vi "String Constant - Through Nested Case Structure.vi"() -> ()   [LabVIEW 2020]
panel:
  in  "OK":bool
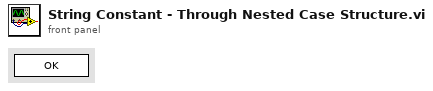
[diagram p1: front panel]
types:
  T1 = enum32{"Invalid", "Standard", "Closed", "Hidden", "Minimized", "Maximized"}
  T2 = enum32{"invalid app kind", "Development System", "Run Time System", "Student Edition", "Embedded LabVIEW", "Evaluation", "Custom"}
  T3 = cluster{"Core":cluster{"Current VI Reference":refnum<vi>, "Close Panel on Exit?":bool}, "Your Boolean data":bool}
  T4 = cluster{"Current VI Reference":refnum<vi>, "Close Panel on Exit?":bool}
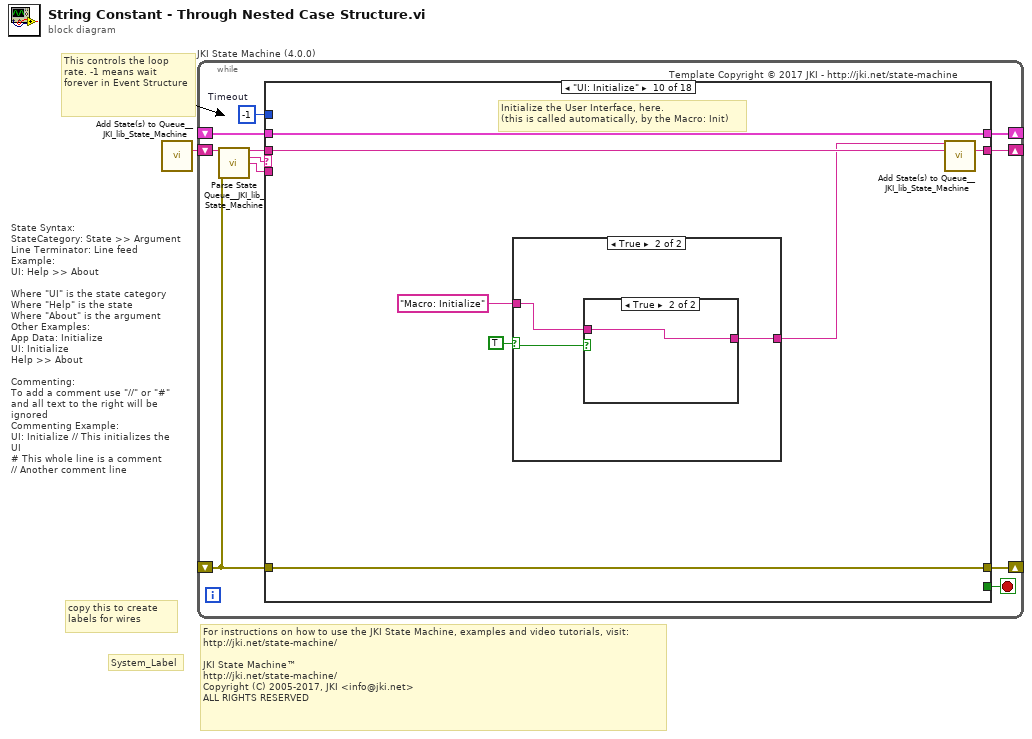
[diagram p0: block diagram]
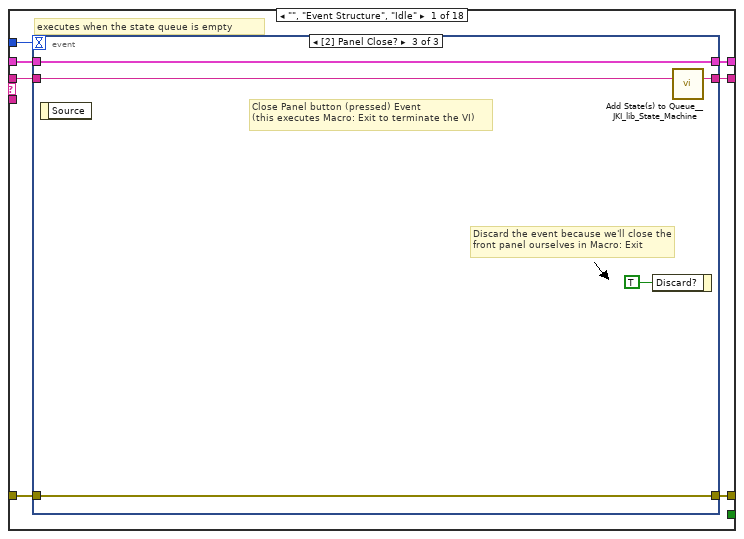
[diagram p2: hidden frame]
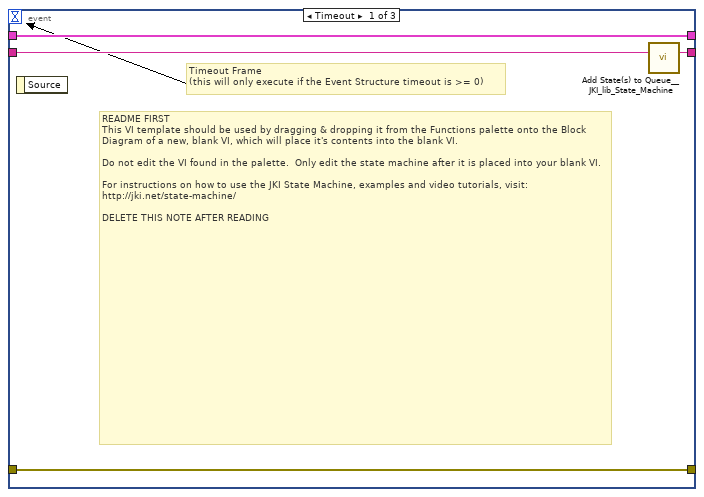
[diagram p3: hidden frame]
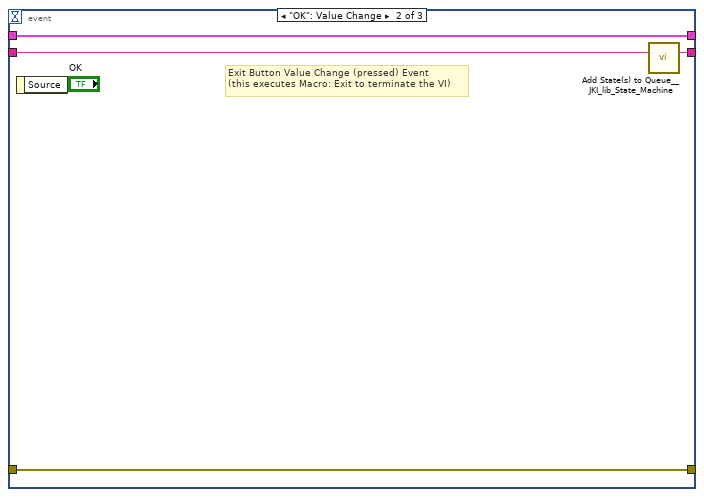
[diagram p4: hidden frame]
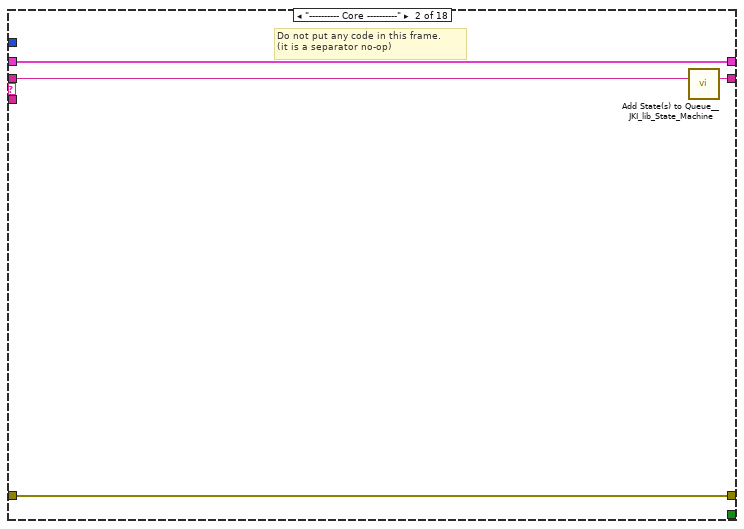
[diagram p5: hidden frame]
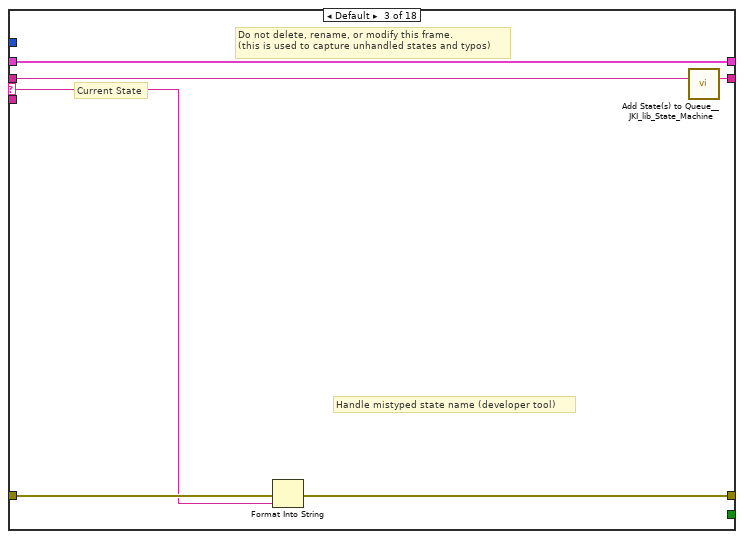
[diagram p6: hidden frame]
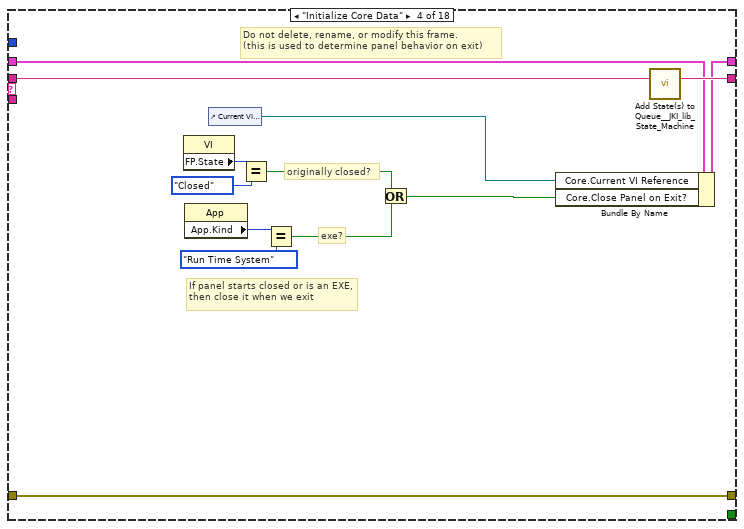
[diagram p7: hidden frame]
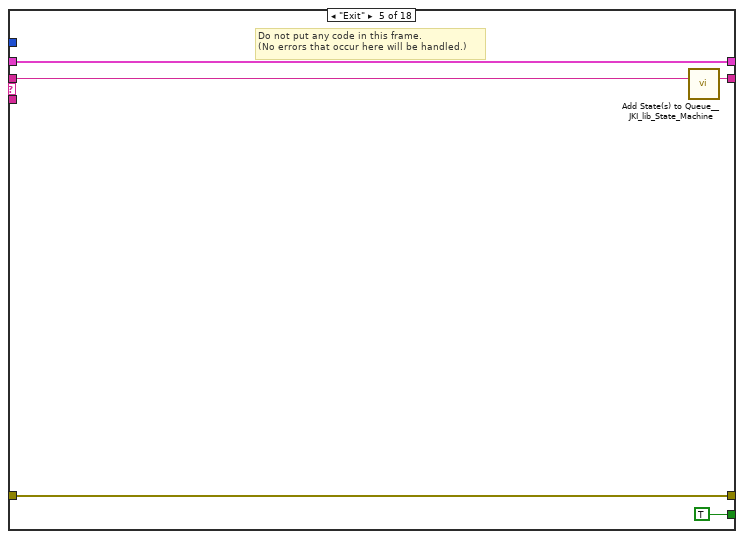
[diagram p8: hidden frame]
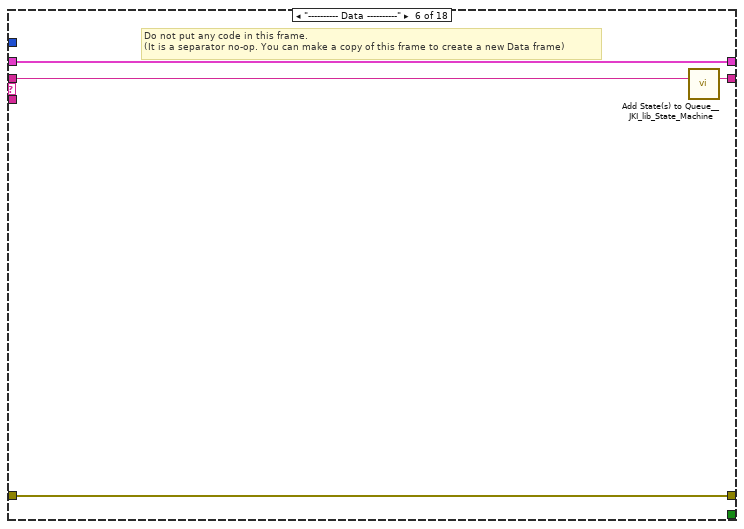
[diagram p9: hidden frame]
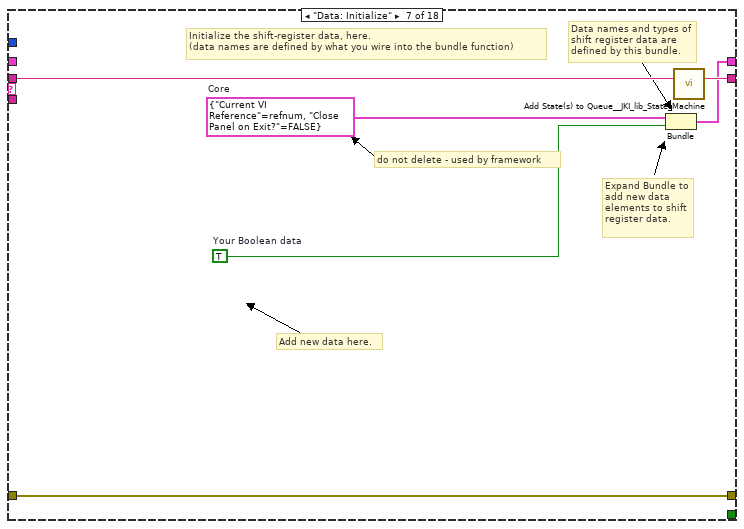
[diagram p10: hidden frame]
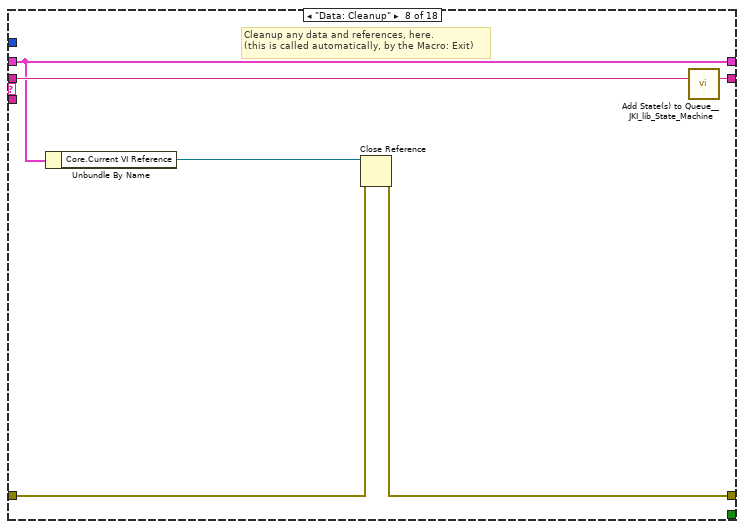
[diagram p11: hidden frame]
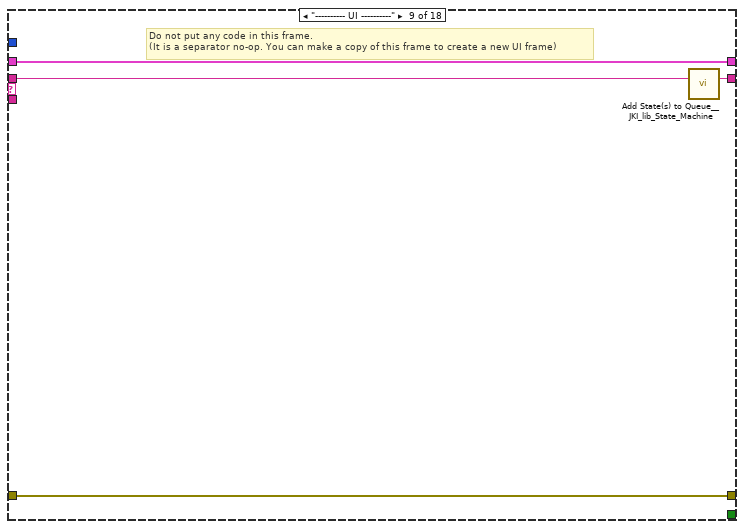
[diagram p12: hidden frame]
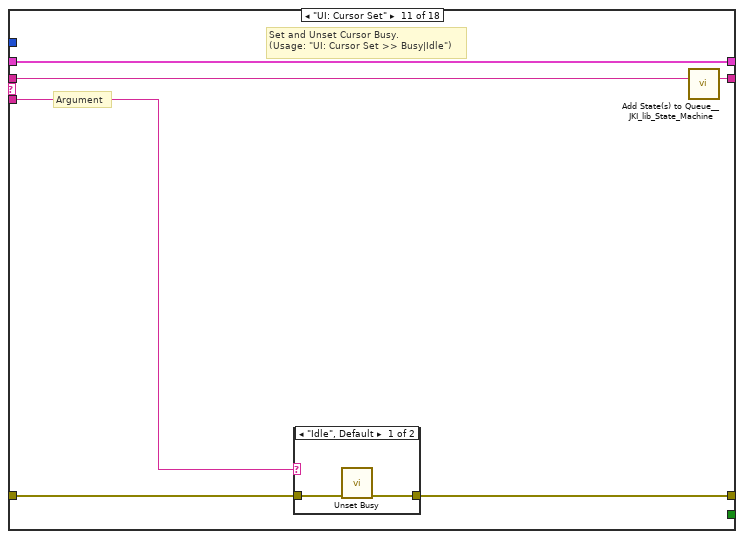
[diagram p15: hidden frame]
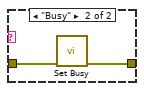
[diagram p16: hidden frame]
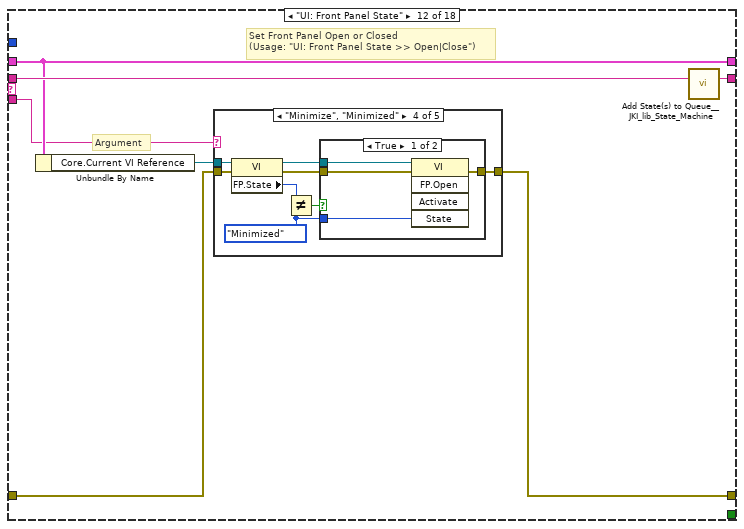
[diagram p17: hidden frame]
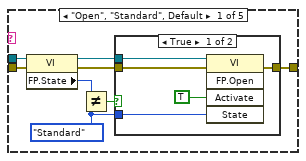
[diagram p18: hidden frame]
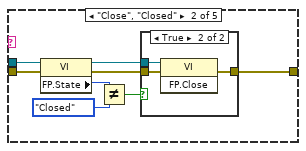
[diagram p20: hidden frame]
diagram:
  # "For instructions on how to use the JKI State Machine, examples and video tutorials, visit:\nhttp://jki.net/state-machine/\n\nJKI State Machine™\nhttp://jki.net/state-machine/\nCopyright (C) 2005-2017, JKI <info@jki.net>\nALL RIGHTS RESERVED"
  # "State Syntax:\nStateCategory: State >> Argument\nLine Terminator: Line feed\nExample:\nUI: Help >> About\n\nWhere \"UI\" is the state category\nWhere \"Help\" is the state\nWhere \"About\" is the argument\nOther Examples:\nApp Data: Initialize\nUI: Initialize\nHelp >> About\n\nCommenting:\nTo add a comment use \"//\" or \"#\" and all text to the right will be ignored\nCommenting Example:\nUI: Initialize // This initializes the UI\n# This whole line is a comment\n// Another comment line"
  # "copy this to create labels for wires"
  # "This controls the loop rate. -1 means wait forever in Event Structure"
  # "System_Label"
  n1 = call <vilib>:"Add State(s) to Queue__JKI_lib_State_Machine.vi"() -> ("States Out"=w1:string)  [unwired: 15 in]
  n2 = while "JKI State Machine (4.0.0)" {
    shift-right: [w5] -> _
    shift-left: _ -> [w4]
    shift-right: [w8] -> _
    shift-left: _ -> [w2]
    shift-right: [w7] -> _
    shift-left: w1 -> [w9]
    stop <- w6 stop-if-true
    w3 = -1  # Timeout
    # "Template Copyright © 2017 JKI - http://jki.net/state-machine"
    n3 = call <vilib>:"Parse State Queue__JKI_lib_State_Machine.vi"("State Queue"=w9, "Error In (no error)"=w2) -> ("Remaining States"=w11:string, "Current State"=w12:string, "Arguments"=w10:string)  [unwired: 11 in]
    n4 = case shown="\"UI: Initialize\"" w12 {
      selector: w12 -> [_ _ w37 _ _ _ _ _ _ _ _ _ _ _ _ _ _ _]
      tunnel: w11 -> [w19 w36 w40 w55 w60 w64 w70 w76 w80 w87 w97 w108 w177 w181 w185 w189 w193 w197]
      tunnel: w10 -> [_ _ _ _ _ _ _ _ _ _ w92 w102 _ _ _ _ _ _]
      tunnel: w4 -> [w17 w33 w38 w48 w58 w61 _ w71 w77 w85 w95 w104 w174 w178 w182 w186 w190 w194]
      tunnel: [w16 w34 w42 w52 w57 w62 w67 w72 w78 w84 w93 w105 w175 w179 w183 w187 w191 w195] -> w8
      tunnel: w2 -> [w15 w34 w41 w52 w57 w62 w67 w73 w78 w84 w94 w106 w175 w179 w183 w187 w191 w195]
      tunnel: [w18 w35 w39 w54 w59 w63 w69 w75 w79 w86 w96 w107 w176 w180 w184 w188 w192 w196] -> w7
      tunnel: [_ _ _ _ TRUE _ _ _ _ _ _ _ _ _ _ _ _ _] -> w6
      tunnel: [w14 w33 w38 w53 w58 w61 w68 w71 w77 w85 w95 w104 w174 w178 w182 w186 w190 w194] -> w5
      tunnel: w3 -> [w13 _ _ _ _ _ _ _ _ _ _ _ _ _ _ _ _ _]
      frame "", "Event Structure", "Idle" {
        # "executes when the state queue is empty"
        n5 = event shown="[2] Panel Close?" {
          selector: _ -> [_ _ _]
          dyn-events: _ -> [_ _ _]
          timeout: w13 -> [_ _ _]
          tunnel: w19 -> [w23 w27 w32]
          tunnel: [w22 w26 w31] -> w18
          tunnel: w17 -> [w20 w24 w29]
          tunnel: [w21 w25 w30] -> w16
          tunnel: w15 -> [w21 w25 w30]
          tunnel: [w20 w24 w29] -> w14
          event Timeout {
            # "README FIRST\nThis VI template should be used by dragging & dropping it from the Functions palette onto the Block Diagram of a new, blank VI, which will place it's contents into the blank VI.\n\nDo not edit the VI found in the palette.  Only edit the state machine after it is placed into your blank VI.\n\nFor instructions on how to use the JKI State Machine, examples and video tutorials, visit:\nhttp://jki.net/state-machine/\n\nDELETE THIS NOTE AFTER READING"
            # "Timeout Frame\n(this will only execute if the Event Structure timeout is >= 0)"
            n6 = event-data() -> ()  [unwired: 1 in, 1 out]
            n7 = call <vilib>:"Add State(s) to Queue__JKI_lib_State_Machine.vi"("State(s) in (\"\")"=w23) -> ("States Out"=w22:string)  [unwired: 14 in]
          }
          event "OK": Value Change {
            # "Exit Button Value Change (pressed) Event\n(this executes Macro: Exit to terminate the VI)"
            n8 = event-data() -> ()  [unwired: 1 in, 1 out]
            n9 = call <vilib>:"Add State(s) to Queue__JKI_lib_State_Machine.vi"("State(s) in (\"\")"=w27) -> ("States Out"=w26:string)  [unwired: 14 in]
          }
          event Panel Close? {
            # "Discard the event because we'll close the front panel ourselves in Macro: Exit"
            # "Close Panel button (pressed) Event\n(this executes Macro: Exit to terminate the VI)"
            n10 = event-data() -> ()  [unwired: 1 in, 1 out]
            n11 = event-data("Discard?"=TRUE) -> ()  [unwired: 1 in, 1 out]
            n12 = call <vilib>:"Add State(s) to Queue__JKI_lib_State_Machine.vi"("State(s) in (\"\")"=w32) -> ("States Out"=w31:string)  [unwired: 14 in]
          }
        }
      }
      frame "---------- Core ----------" {
        # "Do not put any code in this frame.\n(it is a separator no-op)"
        n13 = call <vilib>:"Add State(s) to Queue__JKI_lib_State_Machine.vi"("State(s) in (\"\")"=w36) -> ("States Out"=w35:string)  [unwired: 14 in]
      }
      frame Default {
        # "Current State"
        # "Do not delete, rename, or modify this frame.\n(this is used to capture unhandled states and typos)"
        # "Handle mistyped state name (developer tool)"
        n14 = Format Into String(error in=w41, w37) -> (error out=w42:errorcluster)  [unwired: 2 in, 1 out]
        n15 = call <vilib>:"Add State(s) to Queue__JKI_lib_State_Machine.vi"("State(s) in (\"\")"=w40) -> ("States Out"=w39:string)  [unwired: 14 in]
      }
      frame "Initialize Core Data" {
        # "Do not delete, rename, or modify this frame.\n(this is used to determine panel behavior on exit)"
        # "originally closed?"
        # "exe?"
        # "If panel starts closed or is an EXE, then close it when we exit"
        n16 = property class="VI"() -> ("FP.State"=w45:T1)  [unwired: 2 in, 2 out]
        n17 = property class="App"() -> ("App.Kind"=w51:T2)  [unwired: 2 in, 2 out]
        n18 = control-ref of="Current VI Reference"() -> (w46:refnum<vi>)
        n19 = Equal?(x=w45, y=T1."Closed" ("Front Panel Window:State")) -> (x = y?=w43:bool)
        n20 = Equal?(x=w51, y=T2."Run Time System" ("Application:Kind")) -> (x = y?=w49:bool)
        n21 = Or(x=w43, y=w49) -> (x .or. y?=w47:bool)
        n22 = Bundle By Name(cluster=w48, "Core.Current VI Reference"=w46, "Core.Close Panel on Exit?"=w47) -> (w53:T3)
        n23 = call <vilib>:"Add State(s) to Queue__JKI_lib_State_Machine.vi"("State(s) in (\"\")"=w55) -> ("States Out"=w54:string)  [unwired: 14 in]
      }
      frame "Exit" {
        # "Do not put any code in this frame.\n(No errors that occur here will be handled.)"
        n24 = call <vilib>:"Add State(s) to Queue__JKI_lib_State_Machine.vi"("State(s) in (\"\")"=w60) -> ("States Out"=w59:string)  [unwired: 14 in]
      }
      frame "---------- Data ----------" {
        # "Do not put any code in this frame.\n(It is a separator no-op. You can make a copy of this frame to create a new Data frame)"
        n25 = call <vilib>:"Add State(s) to Queue__JKI_lib_State_Machine.vi"("State(s) in (\"\")"=w64) -> ("States Out"=w63:string)  [unwired: 14 in]
      }
      frame "Data: Initialize" {
        w65 = T4 {"Current VI Reference"=refnum, "Close Panel on Exit?"=FALSE}  # Core
        w66 = TRUE  # Your Boolean data
        # "do not delete - used by framework"
        # "Expand Bundle to add new data elements to shift register data."
        # "Add new data here."
        # "Data names and types of shift register data are defined by this bundle."
        # "Initialize the shift-register data, here.\n(data names are defined by what you wire into the bundle function)"
        n26 = Bundle("Core"=w65, "Your Boolean data"=w66) -> (w68:T3)  [unwired: 1 in]
        n27 = call <vilib>:"Add State(s) to Queue__JKI_lib_State_Machine.vi"("State(s) in (\"\")"=w70) -> ("States Out"=w69:string)  [unwired: 14 in]
      }
      frame "Data: Cleanup" {
        # "Cleanup any data and references, here.\n(this is called automatically, by the Macro: Exit)"
        n28 = Unbundle By Name(w71) -> ("Core.Current VI Reference"=w74:refnum<vi>)
        n29 = Close Reference(reference=w74, error in (no error)=w73) -> (error out=w72:errorcluster)
        n30 = call <vilib>:"Add State(s) to Queue__JKI_lib_State_Machine.vi"("State(s) in (\"\")"=w76) -> ("States Out"=w75:string)  [unwired: 14 in]
      }
      frame "---------- UI ----------" {
        # "Do not put any code in this frame.\n(It is a separator no-op. You can make a copy of this frame to create a new UI frame)"
        n31 = call <vilib>:"Add State(s) to Queue__JKI_lib_State_Machine.vi"("State(s) in (\"\")"=w80) -> ("States Out"=w79:string)  [unwired: 14 in]
      }
      frame "UI: Initialize" {
        # "Initialize the User Interface, here.\n(this is called automatically, by the Macro: Init)"
        n32 = case shown="True" TRUE {
          selector: TRUE -> [_ w89]
          tunnel: [_ w90] -> w83
          tunnel: "Macro: Initialize" -> [_ w88]
          frame False {
          }
          frame True {
            n33 = case shown="True" w89 {
              tunnel: [_ w91] -> w90
              tunnel: w88 -> [_ w91]
              frame False {
              }
              frame True {
              }
            }
          }
        }
        n34 = call <vilib>:"Add State(s) to Queue__JKI_lib_State_Machine.vi"("State(s) in Front (\"\")"=w83, "State(s) in (\"\")"=w87) -> ("States Out"=w86:string)  [unwired: 13 in]
      }
      frame "UI: Cursor Set" {
        # "Argument"
        # "Set and Unset Cursor Busy.\n(Usage: \"UI: Cursor Set >> Busy|Idle\")"
        n35 = case shown="\"Idle\", Default" w92 {
          tunnel: w94 -> [w99 w101]
          tunnel: [w98 w100] -> w93
          frame "Idle", Default {
            n36 = call <vilib>:"Unset Busy.vi"("error in (no error)"=w99) -> ("error out"=w98:errorcluster)  [unwired: 10 in]
          }
          frame "Busy" {
            n37 = call <vilib>:"Set Busy.vi"("error in (no error)"=w101) -> ("error out"=w100:errorcluster)  [unwired: 9 in, 1 out]
          }
        }
        n38 = call <vilib>:"Add State(s) to Queue__JKI_lib_State_Machine.vi"("State(s) in (\"\")"=w97) -> ("States Out"=w96:string)  [unwired: 14 in]
      }
      frame "UI: Front Panel State" {
        # "Argument"
        # "Set Front Panel Open or Closed\n(Usage: \"UI: Front Panel State >> Open|Close\")"
        n39 = Unbundle By Name(w104) -> ("Core.Current VI Reference"=w103:refnum<vi>)
        n40 = case shown="\"Minimize\", \"Minimized\"" w102 {
          tunnel: w106 -> [w114 w129 w140 w153 w166]
          tunnel: [w116 w130 w142 w155 w168] -> w105
          tunnel: w103 -> [w115 w127 w141 w154 w167]
          frame "Open", "Standard", Default {
            w109 = T1."Standard" ("State")
            n41 = property class="VI"(reference=w115, error in=w114) -> (reference out=w112:refnum<vi>, error out=w113:errorcluster, "FP.State"=w111:T1)
            n42 = Not Equal?(x=w111, y=w109) -> (x != y?=w110:bool)
            n43 = case shown="True" w110 {
              tunnel: [w120 w122] -> w116
              tunnel: w113 -> [w119 w122]
              tunnel: w112 -> [w118 _]
              tunnel: w109 -> [w117 _]
              frame True {
                n44 = invoke class="VI" method="FP.Open"(reference=w118, error in=w119, "Activate"=TRUE, "State"=w117) -> (error out=w120:errorcluster)  [unwired: 1 in, 4 out]
              }
              frame False {
              }
            }
          }
          frame "Close", "Closed" {
            n45 = property class="VI"(reference=w127, error in=w129) -> (reference out=w126:refnum<vi>, error out=w128:errorcluster, "FP.State"=w124:T1)
            n46 = Not Equal?(x=w124, y=T1."Closed" ("Front Panel Window:State")) -> (x != y?=w123:bool)
            n47 = case shown="True" w123 {
              tunnel: [w131 w134] -> w130
              tunnel: w128 -> [w131 w133]
              tunnel: w126 -> [_ w132]
              frame False {
              }
              frame True {
                n48 = invoke class="VI" method="FP.Close"(reference=w132, error in=w133) -> (error out=w134:errorcluster)  [unwired: 1 in, 2 out]
              }
            }
          }
          frame "Hidden", "Hide" {
            w135 = T1."Hidden" ("State")
            n49 = property class="VI"(reference=w141, error in=w140) -> (reference out=w138:refnum<vi>, error out=w139:errorcluster, "FP.State"=w137:T1)
            n50 = Not Equal?(x=w137, y=w135) -> (x != y?=w136:bool)
            n51 = case shown="True" w136 {
              tunnel: [w146 w147] -> w142
              tunnel: w139 -> [w145 w147]
              tunnel: w138 -> [w144 _]
              tunnel: w135 -> [w143 _]
              frame True {
                n52 = invoke class="VI" method="FP.Open"(reference=w144, error in=w145, "State"=w143) -> (error out=w146:errorcluster)  [unwired: 2 in, 4 out]
              }
              frame False {
              }
            }
          }
          frame "Minimize", "Minimized" {
            w148 = T1."Minimized" ("State")
            n53 = property class="VI"(reference=w154, error in=w153) -> (reference out=w151:refnum<vi>, error out=w152:errorcluster, "FP.State"=w150:T1)
            n54 = Not Equal?(x=w150, y=w148) -> (x != y?=w149:bool)
            n55 = case shown="True" w149 {
              tunnel: [w159 w160] -> w155
              tunnel: w152 -> [w158 w160]
              tunnel: w151 -> [w157 _]
              tunnel: w148 -> [w156 _]
              frame True {
                n56 = invoke class="VI" method="FP.Open"(reference=w157, error in=w158, "State"=w156) -> (error out=w159:errorcluster)  [unwired: 2 in, 4 out]
              }
              frame False {
              }
            }
          }
          frame "Maximize", "Maximized" {
            w161 = T1."Maximized" ("State")
            n57 = property class="VI"(reference=w167, error in=w166) -> (reference out=w164:refnum<vi>, error out=w165:errorcluster, "FP.State"=w163:T1)
            n58 = Not Equal?(x=w163, y=w161) -> (x != y?=w162:bool)
            n59 = case shown="True" w162 {
              tunnel: [w172 w173] -> w168
              tunnel: w165 -> [w171 w173]
              tunnel: w164 -> [w170 _]
              tunnel: w161 -> [w169 _]
              frame True {
                n60 = invoke class="VI" method="FP.Open"(reference=w170, error in=w171, "State"=w169) -> (error out=w172:errorcluster)  [unwired: 2 in, 4 out]
              }
              frame False {
              }
            }
          }
        }
        n61 = call <vilib>:"Add State(s) to Queue__JKI_lib_State_Machine.vi"("State(s) in (\"\")"=w108) -> ("States Out"=w107:string)  [unwired: 14 in]
      }
      frame "---------- Macro ----------" {
        # "Do not put any code in this frame.\n(It is a separator no-op. You can make a copy of this frame to create a new Macro frame)"
        n62 = call <vilib>:"Add State(s) to Queue__JKI_lib_State_Machine.vi"("State(s) in (\"\")"=w177) -> ("States Out"=w176:string)  [unwired: 14 in]
      }
      frame "Macro: Initialize" {
        # "Initialization Macro\n(This is called once, when the VI starts)"
        n63 = call <vilib>:"Add State(s) to Queue__JKI_lib_State_Machine.vi"("State(s) in (\"\")"=w181) -> ("States Out"=w180:string)  [unwired: 14 in]
      }
      frame "Macro: Exit" {
        # "Exit Macro\n(This is called once, when the VI exits)"
        n64 = call <vilib>:"Add State(s) to Queue__JKI_lib_State_Machine.vi"("State(s) in (\"\")"=w185) -> ("States Out"=w184:string)  [unwired: 14 in]
      }
      frame "---------- New Category ----------" {
        # "Template Separator\n(You can make a copy of, or modify, this frame)"
        n65 = call <vilib>:"Add State(s) to Queue__JKI_lib_State_Machine.vi"("State(s) in (\"\")"=w189) -> ("States Out"=w188:string)  [unwired: 14 in]
      }
      frame "New Category: 1" {
        # "Your code here.\n(You can make a copy of, or modify, this frame)"
        n66 = call <vilib>:"Add State(s) to Queue__JKI_lib_State_Machine.vi"("State(s) in (\"\")"=w193) -> ("States Out"=w192:string)  [unwired: 14 in]
      }
      frame "New Category: 2" {
        # "Your code here.\n(You can make a copy of, or modify, this frame)"
        n67 = call <vilib>:"Add State(s) to Queue__JKI_lib_State_Machine.vi"("State(s) in (\"\")"=w197) -> ("States Out"=w196:string)  [unwired: 14 in]
      }
    }
  }
